vi "create stack writer.vi"(0 "file stub":string, 1 "keyFrameInterval":i32=90, 2 "thresholdAboveBackground":i32=5, 3 "lgDimMinSize":i32=5, 5 "extension":string="mmf", 7 "limit file size?":bool, 9 "maxBytesToWrite":u64=2000000000, 11 "error in (no error)":errorcluster, 12 "anticipated frame rate":dbl=30.0, 14 "smallDimMinSize":i32=3) -> (4 "stack writer pointer":u32, 15 "error out":errorcluster)   [LabVIEW 2013]
uses:
  Image-Stack-Compressor/StackWriterWrapper/LV code/StackWriterWrapper.lvlib
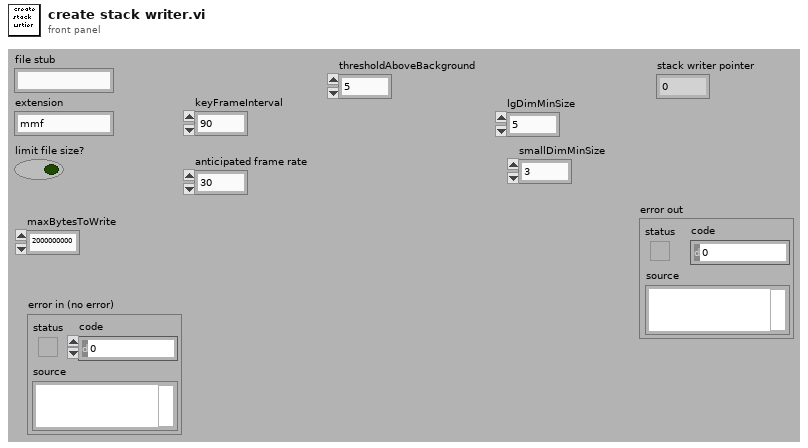
[diagram p1: front panel]
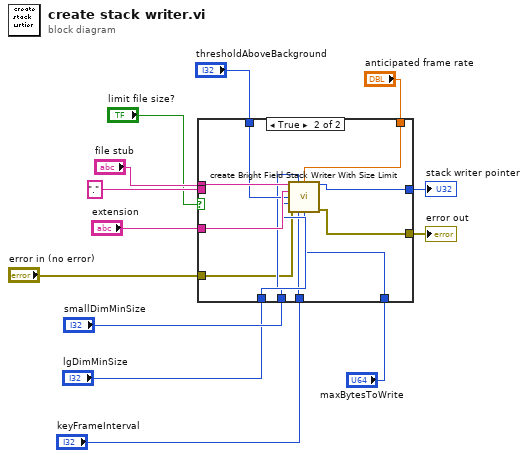
[diagram p0: block diagram]
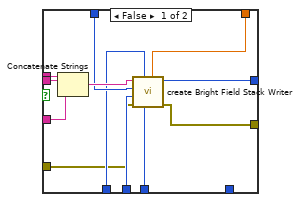
[diagram p2: hidden frame]
diagram:
  n1 = case shown="True" "limit file size?" {
    tunnel: "file stub" -> [w25 w36]
    tunnel: "extension" -> [w24 w35]
    tunnel: "." ("string") -> [w23 _]
    tunnel: "thresholdAboveBackground" -> [w21 w34]
    tunnel: "smallDimMinSize" -> [w20 w31]
    tunnel: "lgDimMinSize" -> [w19 w33]
    tunnel: "keyFrameInterval" -> [w18 w32]
    tunnel: "anticipated frame rate" -> [w17 w28]
    tunnel: [w16 w30] -> w4
    tunnel: [w15 w29] -> w1
    tunnel: "error in (no error)" -> [w14 w27]
    tunnel: "maxBytesToWrite" -> [_ w26]
    frame False {
      n2 = Concatenate Strings(w25, w23, w24) -> (w22:string)
      n3 = call "create Bright Field Stack Writer.vi"("frameRate"=w17, "keyFrameInterval"=w18, "lgDimMinSizem"=w19, "error in (no error)"=w14, "smallDimMinSize"=w20, "thresholdAboveBackground"=w21, "fname"=w22) -> ("error out"=w15:errorcluster, "function return"=w16:u32)  [unwired: 3 in]
    }
    frame True {
      n4 = call "create Bright Field Stack Writer With Size Limit.vi"("fstub"=w36, "lgDimMinSize"=w31, "frameRate"=w28, "ext"=w35, "thresholdAboveBackground"=w34, "smallDimMinSize"=w33, "error in (no error)"=w27, "keyFrameInterval"=w32, "maxBytesToWrite"=w26) -> ("function return"=w30:u32, "error out"=w29:errorcluster)  [unwired: 5 in]
    }
  }
  "stack writer pointer" <- w4
  "error out" <- w1
